vi "Config File (SubVI).vi"(8 "entrée d'erreur (pas d'erreur)":errorcluster, 11 "configuration file path":path=path "C:/Projet_CETAL_DESY_CSCI/POSTES LOCAUX/PROJECT_GAIA_HP/Development/Config/User.ini" caption="chemin du fichier de configuration") -> (0 "sortie d'erreur":errorcluster, 3 "User file contents":dbl[](array[numeric]))   [LabVIEW 2017]
doc: "by Tanguy BOULARD"
uses:
  <vilib>/Utility/config.llb/Read Key (String).vi
  <vilib>/Utility/config.llb/NI_LVConfig.lvlib
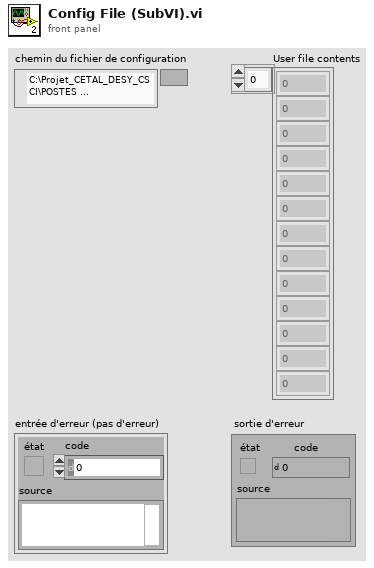
[diagram p1: front panel]
types:
  T1 = typedef "NI_LVConfig.lvlib/Config Data RefNum.ctl" = refnum<k1>
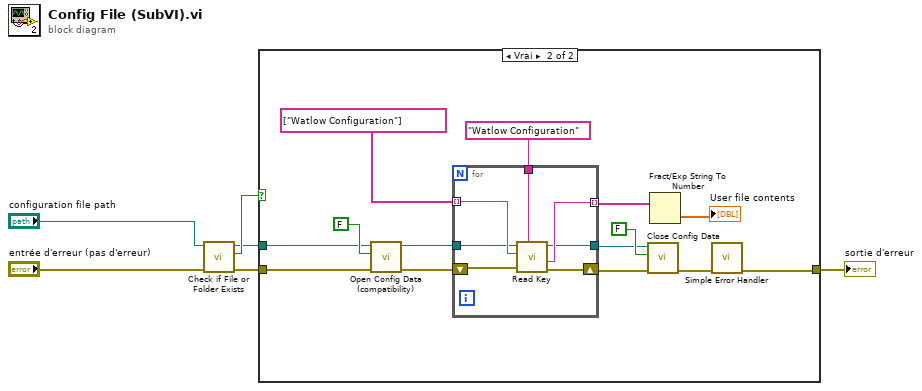
[diagram p0: block diagram]
diagram:
  n1 = call <vilib>:"Check if File or Folder Exists.vi"("error in (no error)"="entrée d'erreur (pas d'erreur)", "path"="configuration file path") -> ("error out"=w3:errorcluster, "file or folder exists?"=w6:bool, "dup path"=w4:path)  [unwired: 7 in]
  n2 = case shown="Vrai" w6 {
    tunnel: w4 -> [_ w17]
    tunnel: w3 -> [w7 w14]
    tunnel: [w7 w12] -> w2
    frame False {
    }
    frame True {
      n3 = call <vilib>:"Open Config Data (compatibility).vi"("error in (no error)"=w14, "create file if necessary (T)"=FALSE ("create file if necessary? (T)"), "configuration file path"=w17) -> ("error out"=w20:errorcluster, "refnum"=w15:T1)  [unwired: 6 in, 1 out]
      n4 = for {
        shift-right: [w27] -> w16
        shift-left: w20 -> [w28]
        tunnel: "Watlow Configuration" ("section") -> [w26]
        tunnel: string[] ["Watlow Configuration"] -> [w25] mode=indexing
        tunnel: w15 -> [w24]
        tunnel: [w23] -> w13 mode=indexing
        tunnel: [w22] -> w11
        n5 = call-poly <vilib>:"Read Key.vi"("section"=w26, "error in (no error)"=w28, "key"=w25, "refnum"=w24) -> ("error out"=w27:errorcluster, "value"=w23:string, "refnum out"=w22:T1)  [unwired: 2 in, 3 out]
      }
      n6 = call <vilib>:"Close Config Data.vi"("error in (no error)"=w16, "write file if changed (T)"=FALSE ("write configuration file? (T)"), "refnum"=w11) -> ("error out"=w19:errorcluster)  [unwired: 8 out]
      n7 = Fract/Exp String To Number(string=w13) -> (number=→"User file contents":dbl[])  [unwired: 3 in, 1 out]
      n8 = call <vilib>:"Simple Error Handler.vi"("error in (no error)"=w19) -> ("error out"=w12:errorcluster)  [unwired: 1 in, 7 out]
    }
  }
  "sortie d'erreur" <- w2
